vi "addToActive.vi"(3 "Baxter in":T2) -> (0 "Active Topics":T1(array[cluster]), 1 "Baxter out":T2)   [LabVIEW 2013]
uses:
  _ROSControl.ctl
  _ROSDirection.ctl
  _ROSDefinition.vi
panel:
  in  "vi reference":refnum<vi>
  in  "error":errorcluster
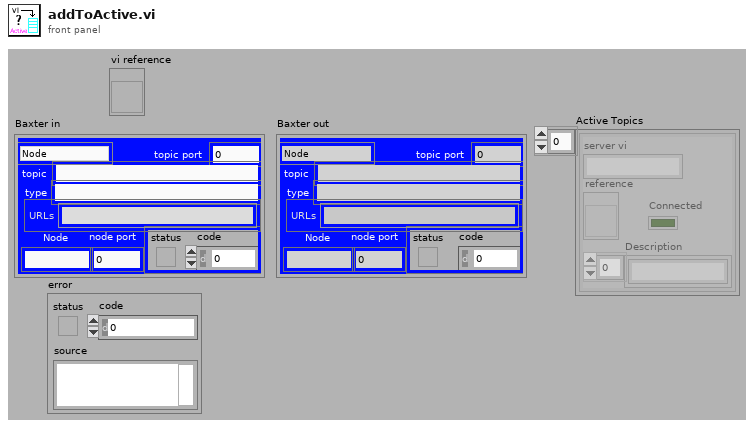
[diagram p1: front panel]
types:
  T1 = cluster{"server vi":string, "reference":refnum<vi>, "Description":string[], "Connected":bool}[]
  T2 = typedef "_ROSControl.ctl" = cluster{"topic port":u16, "Node":string, "topic":string, "type":string, "node port":u32, "error ":errorcluster, "Direction":T3, "APIs":string[]}
  T3 = typedef "_ROSDirection.ctl" = enum16{"Node", "Publisher", "Subscriber", "Service Client"}
  T4 = cluster{"vi name":string, "vi reference":refnum<vi>, string[], bool}
  T5 = cluster{"vi name":string, "vi reference":refnum<vi>, "Description":string[], "Connected":bool}[]
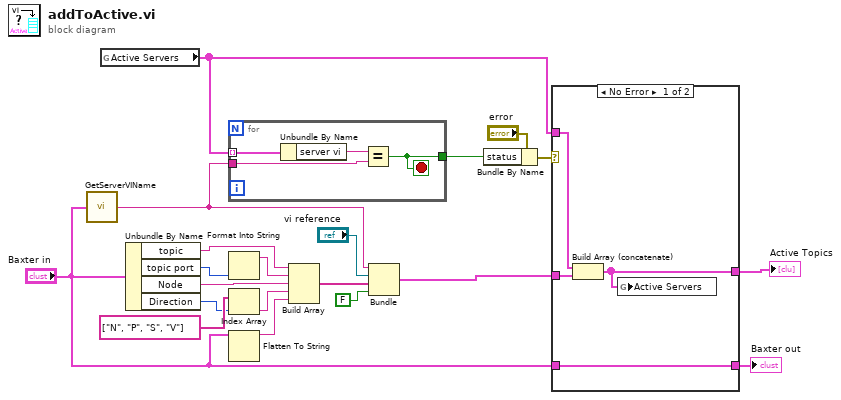
[diagram p0: block diagram]
diagram:
  n1 = call "GetServerVIName.vi"("Baxter"="Baxter in") -> ("vi name"=w6:string)
  n2 = global read "_ROSDefinition.vi" "Active Servers"() -> (w2:T1)
  n3 = Unbundle By Name("Baxter in") -> ("topic"=w11:string, "topic port"=w17:u16, "Node"=w12:string, "Direction"=w14:T3)
  n4 = for {
    tunnel: w2 -> [w24] mode=indexing
    tunnel: w6 -> [w22]
    tunnel: [w21] -> w3
    stop <- w21 stop-if-true
    n5 = Unbundle By Name(w24) -> ("server vi"=w23:string)
    n6 = Equal?(x=w23, y=w22) -> (x = y?=w21:bool)
  }
  n7 = Format Into String(w17) -> (resulting string=w16:string)  [unwired: 3 in, 1 out]
  n8 = Index Array(array=string[] ["N", "P", "S", "V"], index=w14) -> (element=w13:string)
  n9 = Flatten To String(anything="Baxter in") -> (data string=w7:string)  [unwired: 3 in, 2 out]
  n10 = Build Array(w11, w16, w12, w13, w7) -> (w10:string[])
  n11 = Bundle("vi name"=w6, "vi reference"="vi reference", w10, FALSE) -> (w18:T4)  [unwired: 1 in]
  n12 = Bundle By Name(cluster="error", "status"=w3) -> (w4:errorcluster)
  n13 = case shown="No Error" w4 {
    tunnel: [w27 w30] -> w20
    tunnel: "Baxter in" -> [w27 w30]
    tunnel: w18 -> [w28 _]
    tunnel: [w26 w29] -> w9
    tunnel: w2 -> [w25 w29]
    frame No Error {
      n14 = Build Array (concatenate)(w25, w28) -> (w26:T5)
      n15 = global write "_ROSDefinition.vi" "Active Servers"(w26) -> ()
    }
    frame Error {
    }
  }
  "Baxter out" <- w20
  "Active Topics" <- w9
